vi "Check Errors If Full.vi"(8 "error in (no error)":errorcluster, 11 "VisaComms in":refnum<class "VisaComms.lvclass">) -> (0 "error out":errorcluster, 3 "VisaComms out":refnum<class "VisaComms.lvclass">)   [LabVIEW 2020, in "CTI.lvlib" / "VisaComms.lvclass"]
uses:
  VisaComms.lvclass
  Error Reporting.ctl
  VisaComms.lvclass/VisaComms.ctl
  CTI.lvlib
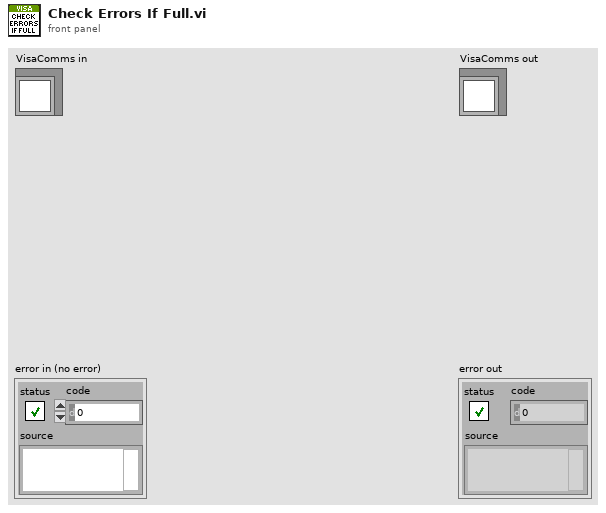
[diagram p1: front panel]
types:
  T1 = typedef "CTI.lvlib/Error Reporting.ctl" = enum16{"Minimal", "Moderate", "Full"}
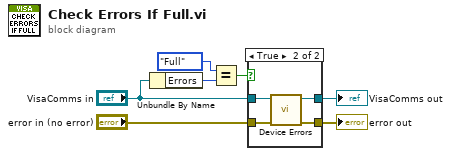
[diagram p0: block diagram]
diagram:
  n1 = Unbundle By Name("VisaComms in") -> ("Errors"=w7:T1)
  n2 = Equal?(x=Error_Reporting."Full", y=w7) -> (x = y?=w3:bool)
  n3 = case shown="True" w3 {
    tunnel: "VisaComms in" -> [w9 w13]
    tunnel: "error in (no error)" -> [w8 w12]
    tunnel: [w9 w11] -> w2
    tunnel: [w8 w10] -> w1
    frame False {
    }
    frame True {
      n4 = call-dynamic "Device Errors.vi"("error in (no error)"=w12, "VisaComms in"=w13) -> ("error out"=w10:errorcluster, "VisaComms out"=w11:refnum<class "VisaComms.lvclass">)  [unwired: 8 in]
    }
  }
  "error out" <- w1
  "VisaComms out" <- w2
